vi "sv_Align Waveform (N Channels).vi"(0 "waveforms":waveform(dbl)[](array[waveform]), 2 "reset?":bool, 5 "filtered waveforms":waveform(dbl)[](array[waveform])) -> (4 "waveforms out":waveform(dbl)[](array[waveform]), 6 "filtered waveforms out":waveform(dbl)[](array[waveform]), 8 "residue waveforms":waveform(dbl)[](array[waveform]))   [LabVIEW 2017, in "SoundVib_ContSweptSine.lvlib"]
uses:
  <vilib>/addons/Sound and Vibration/svt_Continuous Swept Sine/SoundVib_ContSweptSine.lvlib
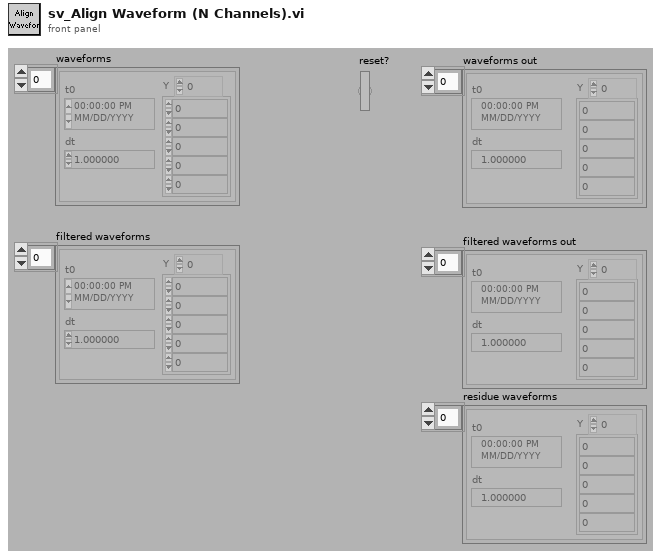
[diagram p1: front panel]
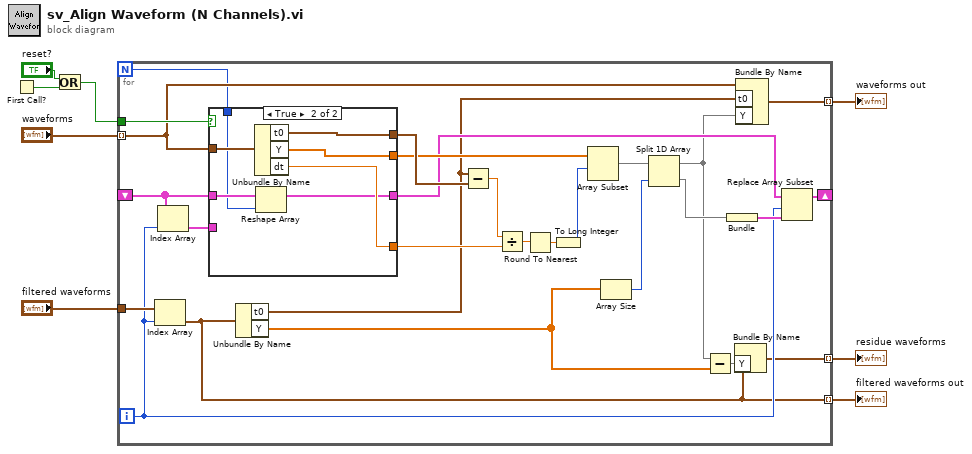
[diagram p0: block diagram]
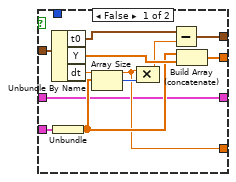
[diagram p2: hidden frame]
diagram:
  n1 = First Call?() -> (First Call?: T/F=w7:bool)
  n2 = Or(x="reset?", y=w7) -> (x .or. y?=w6:bool)
  n3 = for {
    N -> [w9]
    shift-right: [w22] -> _
    shift-left: _ -> [w33]
    tunnel: w6 -> [w34]
    tunnel: "waveforms" -> [w10] mode=indexing
    tunnel: "filtered waveforms" -> [w16]
    tunnel: [w20] -> w4 mode=indexing
    tunnel: [w14] -> w3 mode=indexing
    tunnel: [w11] -> w2 mode=indexing
    i -> [w15]
    n4 = Index Array(array=w16, index=w15) -> (element=w14:waveform(dbl))
    n5 = Index Array(array=w33, index=w15) -> (element=w35:cluster{dbl[]})
    n6 = case shown="True" w34 {
      tunnel: w10 -> [w45 w50]
      tunnel: w35 -> [w46 _]
      tunnel: w33 -> [w36 w49]
      tunnel: [w43 w53] -> w27
      tunnel: [w38 w52] -> w32
      tunnel: [w37 w51] -> w30
      tunnel: [w36 w47] -> w21
      tunnel: w9 -> [_ w48]
      frame False {
        n7 = Unbundle By Name(w45) -> ("t0"=w40:timestamp, "Y"=w44:dbl[], "dt"=w37:dbl)
        n8 = Unbundle(w46) -> (w42:dbl[])
        n9 = Array Size(array=w42) -> (size(s)=w41:i32)
        n10 = Compound Arithmetic op=MULTIPLY(w37, w41) -> (w39:dbl)
        n11 = Subtract(x=w40, y=w39) -> (x-y=w38:timestamp)
        n12 = Build Array (concatenate)(w42, w44) -> (w43:dbl[])
      }
      frame True {
        n13 = Unbundle By Name(w50) -> ("t0"=w52:timestamp, "Y"=w53:dbl[], "dt"=w51:dbl)
        n14 = Reshape Array(w49, w48) -> (w47:cluster{dbl[]}[])
      }
    }
    n15 = Unbundle By Name(w14) -> ("t0"=w17:timestamp, "Y"=w19:dbl[])
    n16 = Subtract(x=w17, y=w32) -> (x-y=w31:dbl)
    n17 = Divide(x=w31, y=w30) -> (x/y=w29:dbl)
    n18 = Round To Nearest(number=w29) -> (nearest integer value=w28:dbl)
    n19 = To Long Integer(number=w28) -> (32bit integer=w26:i32)
    n20 = Array Subset(array=w27, index=w26) -> (w25:dbl[])  [unwired: 1 in]
    n21 = Array Size(array=w19) -> (size(s)=w18:i32)
    n22 = Split 1D Array(array=w25, index=w18) -> (first subarray=w12:dbl[], second subarray=w24:dbl[])
    n23 = Subtract(x=w12, y=w19) -> (x-y=w13:dbl[])
    n24 = Bundle(w24) -> (w23:cluster{dbl[]})  [unwired: 1 in]
    n25 = Bundle By Name(cluster=w14, "Y"=w13) -> (w11:waveform(dbl))
    n26 = Bundle By Name(cluster=w10, "t0"=w17, "Y"=w12) -> (w20:waveform(dbl))
    n27 = Replace Array Subset(array=w21, new element=w23, index=w15) -> (w22:cluster{dbl[]}[])
  }
  "waveforms out" <- w4
  "filtered waveforms out" <- w3
  "residue waveforms" <- w2
